vi "[GV]_SPEED1.vi"() -> ()   [LabVIEW 2016]
panel:
  in  "SPEED1":u16
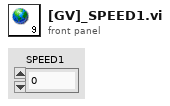
[diagram p1: front panel]
diagram:
